vi "Main.vi"() -> ()   [LabVIEW 2018]
uses:
  Ctl/State.ctl
  Ctl/TriggerType.ctl
  Ctl/AO Channel.ctl
  <vilib>/DAQmx/write.llb/DAQmx Write (Digital 1D Bool NChan 1Samp 1Line).vi
  <vilib>/DAQmx/read.llb/DAQmx Read (Digital 1D Bool NChan 1Samp 1Line).vi
  <vilib>/DAQmx/read.llb/DAQmx Read (Analog 1D DBL NChan 1Samp).vi
  <vilib>/DAQmx/write.llb/DAQmx Write (Analog 1D DBL NChan 1Samp).vi
  <vilib>/DAQmx/miscellaneous.llb/DAQmx Fill In Error Info.vi
  Global Variable/StorageAcquireData.vi
panel:
  out "不响应修改预设波形":bool
  out "电流方向":string
  in  "电流反向输出":bool
  in  "电流正向输出":bool=TRUE
  out "电流方向开关输出":bool[](array[boolean])
  out "数字信号错误输出":errorcluster
  in  "数字输出通道参数设置":T1={"数据输出通道设置"={"lines"="", "line grouping"=1}, "采样设置"={"rate"=1000.0, "sample mode"=10178, "samples per channel"=1000}, "ConvLateErrorsToWarnings"=FALSE} {"采样设置"."sample mode" items=["Finite Samples"=10178, "Continuous Samples"=10123, "Hardware Timed Single Point"=12522]; "采样设置"."rate" format="%0.2f"; "数据输出通道设置"."line grouping" items=["one channel for each line", "one channel for all lines"]}
  in  "DAQ数字采集通道参数设置":T2={"数据采集设置"={"lines"="", "line grouping"=1}, "采样设置"={"rate"=1000.0, "sample mode"=10178, "samples per channel"=1000}, "ConvLateErrorsToWarnings"=FALSE} {"采样设置"."sample mode" items=["Finite Samples"=10178, "Continuous Samples"=10123, "Hardware Timed Single Point"=12522]; "采样设置"."rate" format="%0.2f"; "数据采集设置"."line grouping" items=["one channel for each line", "one channel for all lines"]}
  in  "模拟输出通道设置":T3={"数据输出通道设置"={"maximum value"=5.0, "minimum value"=-5.0, "input terminal configuration"=-1, "physical channels"=""}, "采样设置"={"rate"=1000.0, "sample mode"=10178, "samples per channel"=1000}, "ConvLateErrorsToWarnings"=FALSE} {"采样设置"."sample mode" items=["Finite Samples"=10178, "Continuous Samples"=10123, "Hardware Timed Single Point"=12522]; "采样设置"."rate" format="%0.2f"; "数据输出通道设置"."input terminal configuration" items=["Default"=-1, "RSE"=10083, "NRSE"=10078, "Differential"=10106, "Pseudodifferential"=12529]; "数据输出通道设置"."minimum value" format="%0.2f"; "数据输出通道设置"."maximum value" format="%0.2f"}
  in  "DAQ模拟采集通道参数设置":T4={"数据采集通道设置"={"physical channels"="", "maximum value"=5.0, "minimum value"=-5.0, "input terminal configuration"=-1}, "采样设置"={"rate"=1000.0, "sample mode"=10178, "samples per channel"=1000}, "ConvLateErrorsToWarnings"=FALSE} {"采样设置"."sample mode" items=["Finite Samples"=10178, "Continuous Samples"=10123, "Hardware Timed Single Point"=12522]; "采样设置"."rate" format="%0.2f"; "数据采集通道设置"."input terminal configuration" items=["Default"=-1, "RSE"=10083, "NRSE"=10078, "Differential"=10106, "Pseudodifferential"=12529]; "数据采集通道设置"."minimum value" format="%0.2f"; "数据采集通道设置"."maximum value" format="%0.2f"}
  out "预设电流波形":cluster{"xi used":dbl[], "yi":dbl[]}(graph)
  out "插值后输出波形幅值":dbl[](array[numeric])
  in  "修改波形参数":T5
  in  "导入导出波形文件":T6
  in  "预设波形数组":dbl[][](array[numeric])
  out "波形解析成功":bool
  in  "一炮最长运行时间点（ms)":dbl
  in  "PID 参数":T7={"proportional gain (Kc)"=1.0, "integral time (Ti, min)"=0.01, "derivative time (Td, min)"=0.0} {"derivative time (Td, min)" format="%.3f"; "integral time (Ti, min)" format="%.3f"; "proportional gain (Kc)" format="%.3f"}
  in  "触发时间":dbl
  out "模拟信号错误":errorcluster caption="模拟信号错误输出"
  in  "READY_COLD_TO_HOT":bool=TRUE
  out "电源下一个状态":T8
  out "程序停止":bool
  in  "停止":bool
  in  "外部故障":bool
  out "故障状态指示":cluster{"模拟信号故障？":bool, "数字信号故障？":bool}
  in  "模拟保护信号设定值":cluster{"设定值":dbl, "保护配置规则":bool}
  in  "触发参数设置":cluster{"枚举":T9, "触发基准电平":dbl}
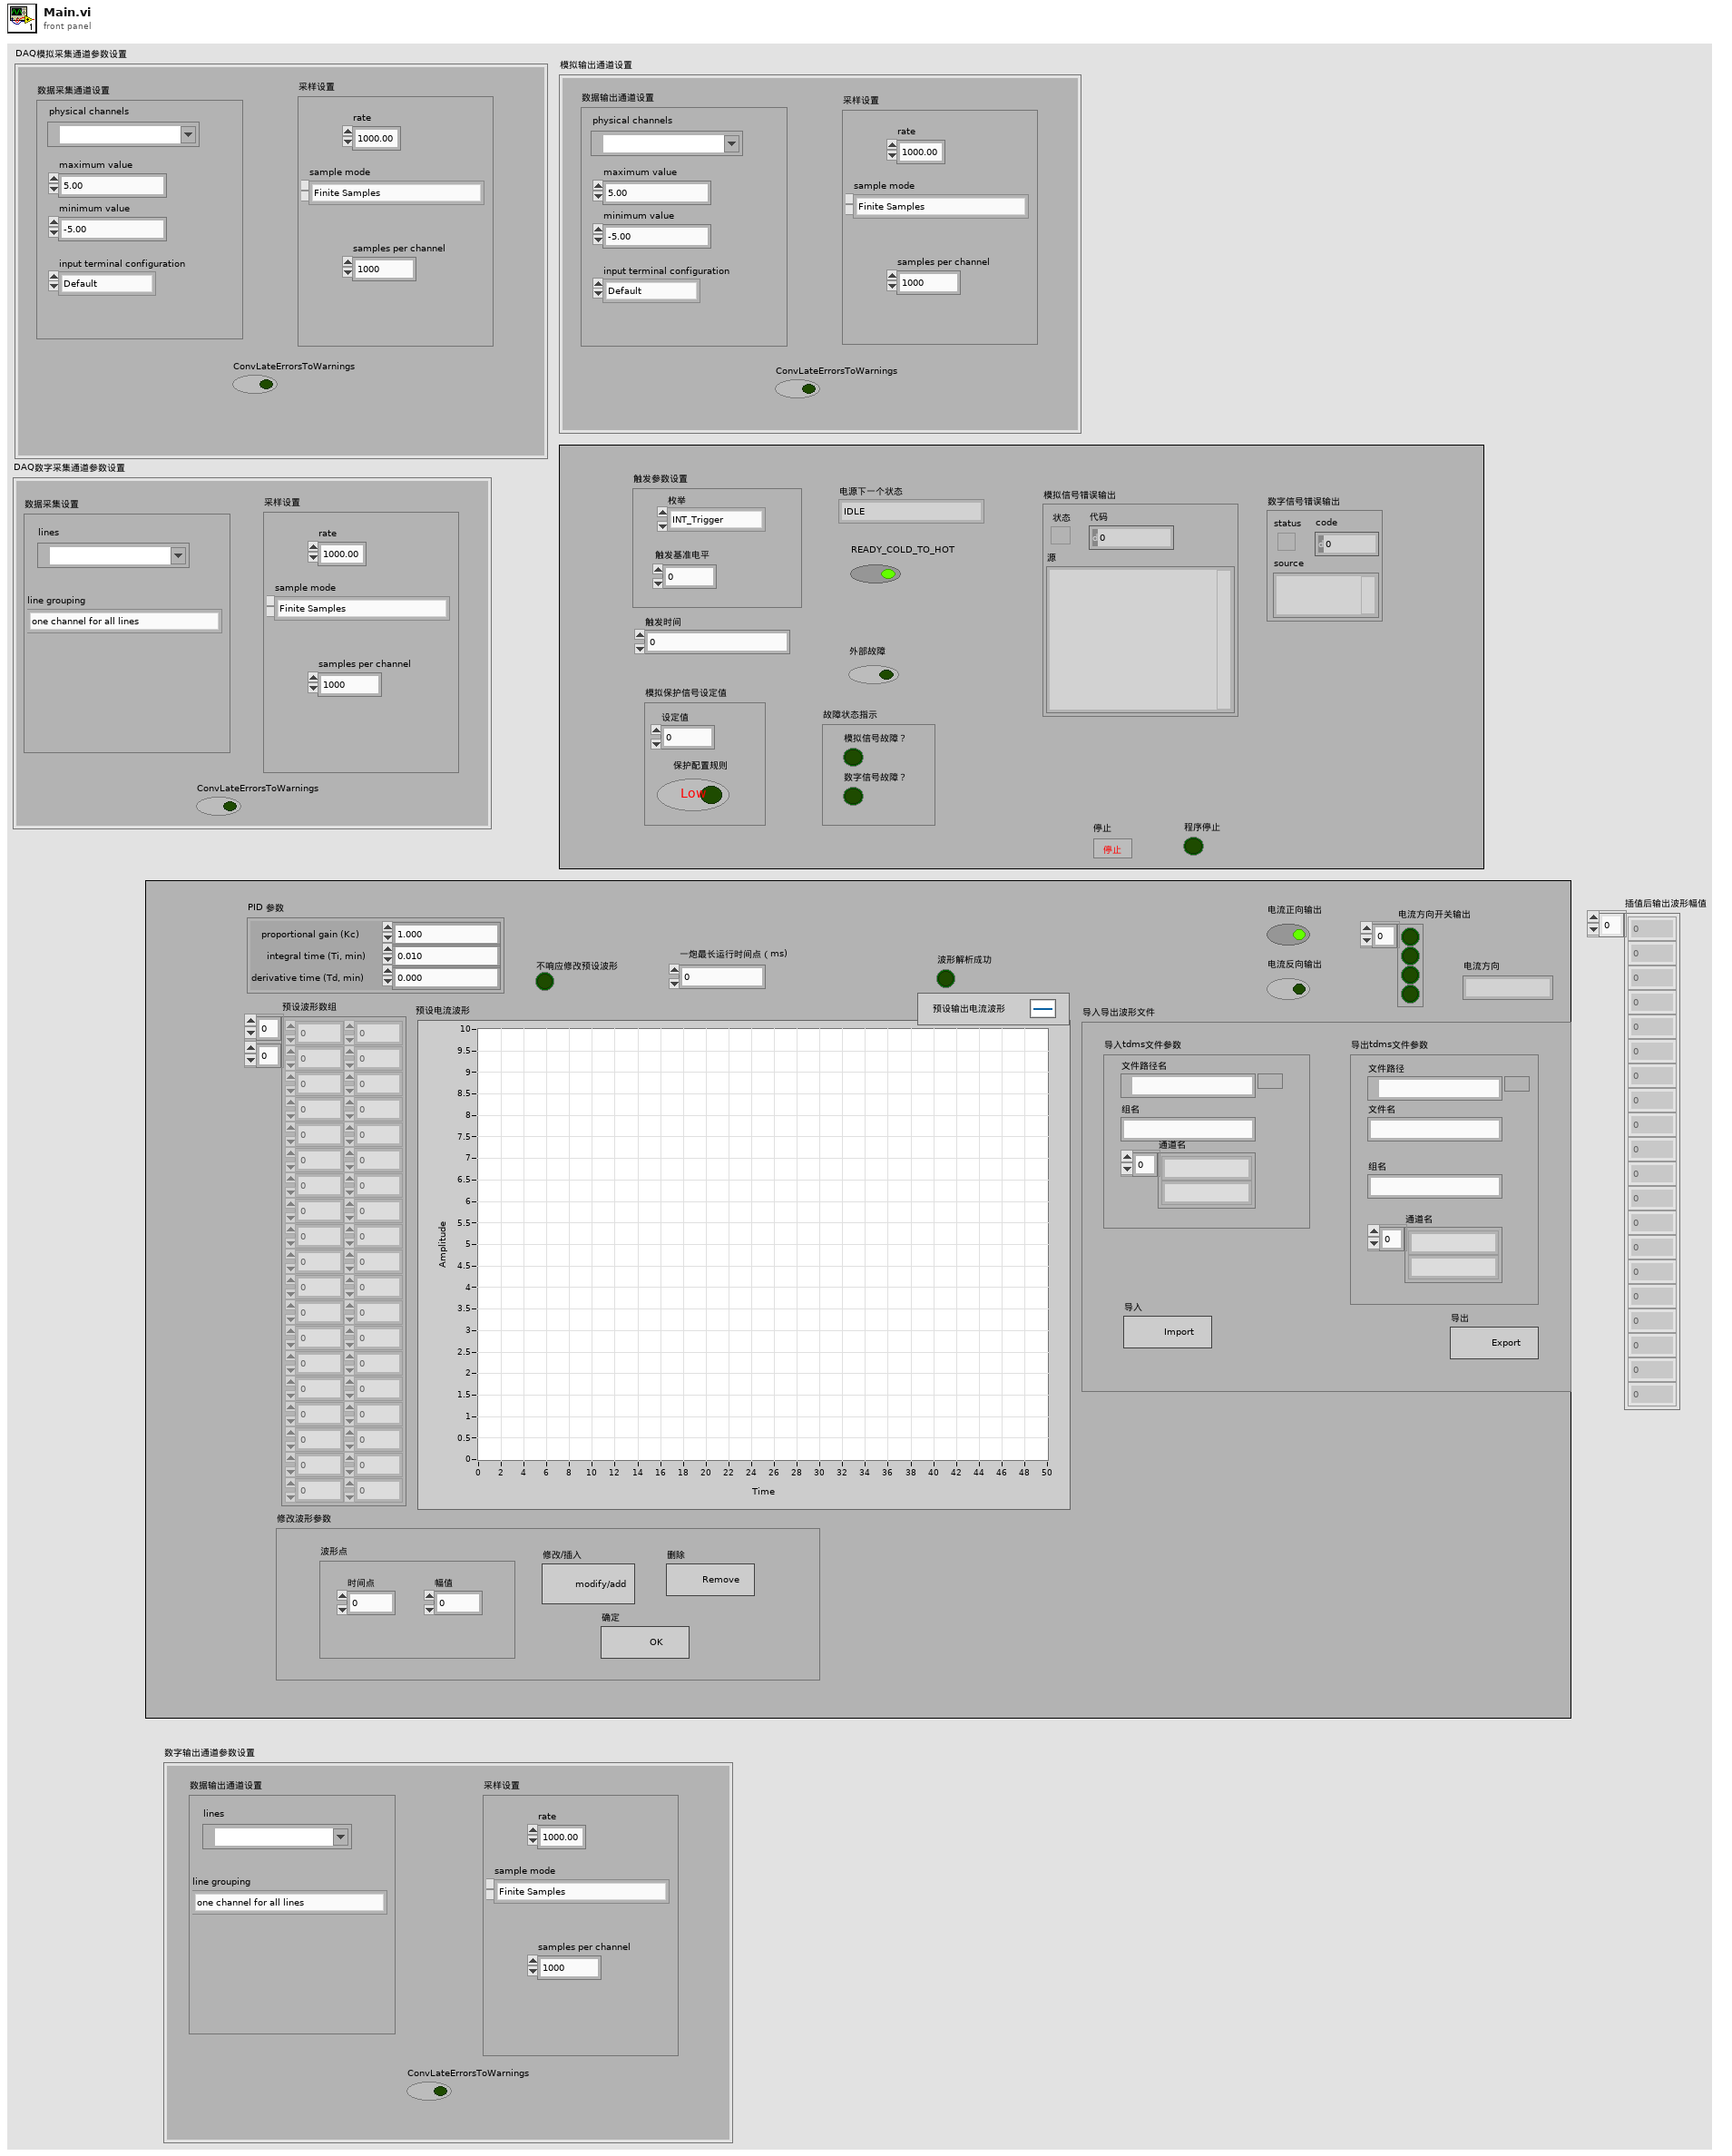
[diagram p1: front panel]
types:
  T1 = cluster{"数据输出通道设置":cluster{"lines":tag, "line grouping":i32}, "采样设置":cluster{"rate":dbl, "sample mode":i32, "samples per channel":i32}, "ConvLateErrorsToWarnings":bool}
  T2 = cluster{"数据采集设置":cluster{"lines":tag, "line grouping":i32}, "采样设置":cluster{"rate":dbl, "sample mode":i32, "samples per channel":i32}, "ConvLateErrorsToWarnings":bool}
  T3 = cluster{"数据输出通道设置":cluster{"maximum value":dbl, "minimum value":dbl, "input terminal configuration":i32, "physical channels":tag}, "采样设置":cluster{"rate":dbl, "sample mode":i32, "samples per channel":i32}, "ConvLateErrorsToWarnings":bool}
  T4 = cluster{"数据采集通道设置":cluster{"physical channels":tag, "maximum value":dbl, "minimum value":dbl, "input terminal configuration":i32}, "采样设置":cluster{"rate":dbl, "sample mode":i32, "samples per channel":i32}, "ConvLateErrorsToWarnings":bool}
  T5 = cluster{"波形点":cluster{"时间点":dbl, "幅值":dbl}, "修改/插入":bool, "删除":bool, "确定":bool}
  T6 = cluster{"导出tdms文件参数":cluster{"组名":string, "通道名":string[], "文件路径":path, "文件名":string}, "导入tdms文件参数":cluster{"文件路径名":path, "组名":string, "通道名":string[]}, "导入":bool, "导出":bool}
  T7 = cluster{"proportional gain (Kc)":dbl, "integral time (Ti, min)":dbl, "derivative time (Td, min)":dbl}
  T8 = typedef "State.ctl" = enum16{"IDLE", "READY_COLD", "READY_HOT", "RUN", "ERROR"}
  T9 = typedef "TriggerType.ctl" = enum16{"INT_Trigger", "Ext_Trigger"}
  T10 = typedef "AO Channel.ctl" = enum16{"启用1个输出通道", "启用2个输出通道", "启用3个输出通道", "启用4个输出通道", "启用5个输出通道", "启用6个输出通道", "启用7个输出通道", "启用8个输出通道"}
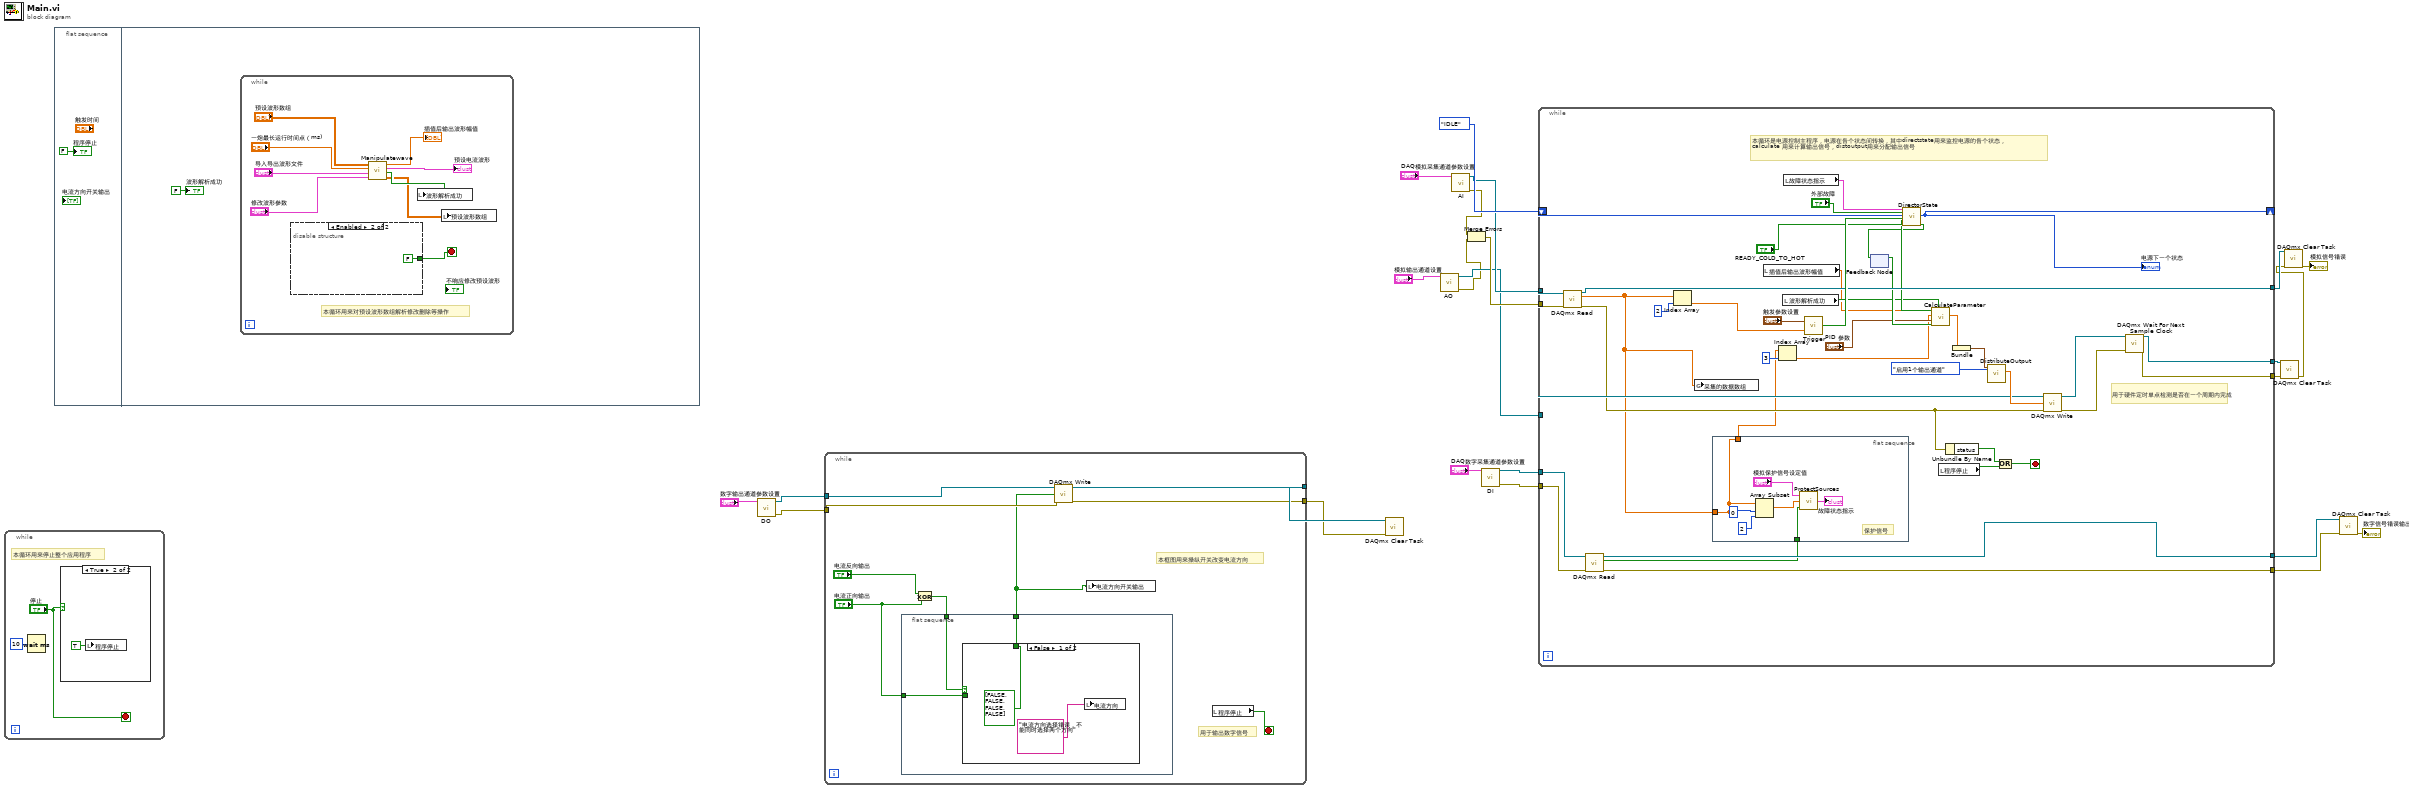
[diagram p0: block diagram]
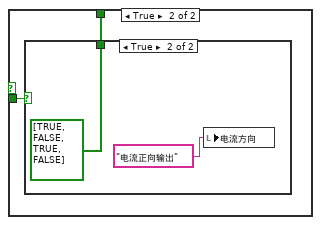
[diagram p2: hidden frame]
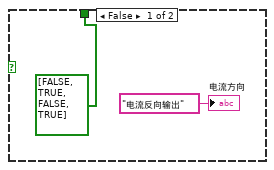
[diagram p3: hidden frame]
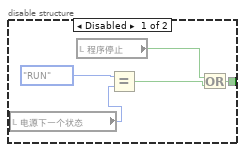
[diagram p4: hidden frame]
diagram:
  n1 = while {
    stop <- "停止" stop-if-true
    # "本循环用来停止整个应用程序"
    n2 = Wait (ms)(milliseconds to wait=u32 10) -> ()  [unwired: 1 out]
    n3 = case shown="True" "停止" {
      frame False {
      }
      frame True {
        n4 = local write "程序停止"(TRUE ("布尔")) -> ()
      }
    }
  }
  n5 = flat-sequence {
    frame #0 {
      "程序停止" <- FALSE ("布尔")
    }
    frame #1 {
      n6 = while {
        stop <- w31 stop-if-true
        # "本循环用来对预设波形数组解析修改删除等操作"
        n7 = disable-structure shown="Enabled" {
          disable-tunnel: [w39 FALSE] -> w31
          frame Disabled {
            n8 = local read "电源下一个状态"() -> (w43:T8)
            n9 = local read "程序停止"() -> (w41:bool)
            n10 = Equal?(x=State."RUN" ("电源状态"), y=w43) -> (x = y?=w40:bool)
            n11 = Or(x=w41, y=w40) -> (x .or. y?=w39:bool)
          }
          frame Enabled {
          }
        }
        n12 = call "Manipulatewave.vi"("修改波形参数"="修改波形参数", "导入导出波形文件"="导入导出波形文件", "一炮最长运行时间点（ms)"="一炮最长运行时间点（ms)", "预设波形数组"="预设波形数组") -> ("波形数组"=w30:dbl[][], "波形解析正确"=w32:bool, "XY Graph"=→"预设电流波形":cluster{"xi used":dbl[], "yi":dbl[]}, "插值后输出波形幅值"=→"插值后输出波形幅值":dbl[])  [unwired: 4 in]
        n13 = local write "波形解析成功"(w32) -> ()
        n14 = local write "预设波形数组"(w30) -> ()
      }
      "波形解析成功" <- FALSE ("波形解析成功")
    }
  }
  n15 = call "DO.vi"("数字输出通道参数设置"="数字输出通道参数设置") -> ("error out"=w1:errorcluster, "task out"=w2:refnum<k21>)  [unwired: 9 in]
  n16 = while {
    tunnel: [w52] -> w4
    tunnel: [w51] -> w3
    tunnel: w2 -> [w50]
    tunnel: w1 -> [w49]
    stop <- w53 stop-if-true
    # "本框图用来操纵开关改变电流方向"
    # "用于输出数字信号"
    n17 = flat-sequence {
      tunnel: w47 -> [w56]
      tunnel: "电流正向输出" -> [w55]
      tunnel: [w54] -> w45
      frame #0 {
        n18 = case shown="False" w56 {
          tunnel: w55 -> [_ w60]
          tunnel: [bool[] [FALSE, FALSE, FALSE, FALSE] ("电流方向开关输出") w59] -> w54
          frame False {
            n19 = local write "电流方向"("电流方向选择错误，不能同时选择两个方向" ("电流方向")) -> ()
          }
          frame True {
            n20 = case shown="True" w60 {
              tunnel: [bool[] [FALSE, TRUE, FALSE, TRUE] ("电流方向开关输出") bool[] [TRUE, FALSE, TRUE, FALSE] ("电流方向开关输出")] -> w59
              frame False {
                "电流方向" <- "电流反向输出" ("电流方向")
              }
              frame True {
                n21 = local write "电流方向"("电流正向输出" ("电流方向")) -> ()
              }
            }
          }
        }
      }
    }
    n22 = Exclusive Or(1:"电流正向输出", 2:"电流反向输出") -> (0:w47:bool)
    n23 = call-poly <vilib>:"DAQmx Write.vi"("task/channels in"=w50, "data"=w45, "error in"=w49) -> ("task out"=w52:refnum<k21>, "error out"=w51:errorcluster)  [unwired: 10 in, 1 out]
    n24 = local write "电流方向开关输出"(w45) -> ()
    n25 = local read "程序停止"() -> (w53:bool)
  }
  n26 = call <vilib>:"DAQmx Clear Task.vi"("task in"=w4, "error in"=w3) -> ()  [unwired: 13 in, 1 out]
  n27 = call "AO.vi"("模拟输出通道设置"="模拟输出通道设置") -> ("error out"=w12:errorcluster, "task out"=w13:refnum<k21>)  [unwired: 8 in]
  n28 = call "AI.vi"("DAQ模拟采集通道参数设置"="DAQ模拟采集通道参数设置") -> ("error out"=w16:errorcluster, "task out"=w15:refnum<k21>)  [unwired: 8 in]
  n29 = Merge Errors(w16, w12) -> (w23:errorcluster)
  n30 = call "DI.vi"("DAQ数字采集通道参数设置"="DAQ数字采集通道参数设置") -> ("error out"=w9:errorcluster, "task out"=w10:refnum<k21>)  [unwired: 9 in]
  n31 = while {
    shift-right: [w103] -> _
    shift-left: State."IDLE" ("电源状态") -> [w104]
    tunnel: w15 -> [w99]
    tunnel: w23 -> [w98]
    tunnel: w13 -> [w89]
    tunnel: [w86] -> w22
    tunnel: [w85] -> w21
    tunnel: [w84] -> w20
    tunnel: w10 -> [w69]
    tunnel: w9 -> [w68]
    tunnel: [w67] -> w8
    tunnel: [w65] -> w7
    stop <- w102 stop-if-true
    # "用于硬件定时单点检测是否在一个周期内完成"
    # "本循环是电源控制主程序，电源在各个状态间转换，其中directstate用来监控电源的各个状态，\ncalculate 用来计算输出信号，distoutput用来分配输出信号"
    n32 = call-poly <vilib>:"DAQmx Read.vi"("task/channels in"=w99, "error in"=w98) -> ("task out"=w84:refnum<k21>, "data"=w70:dbl[], "error out"=w83:errorcluster)  [unwired: 11 in]
    n33 = call-poly <vilib>:"DAQmx Read.vi"("task/channels in"=w69, "error in"=w68) -> ("task out"=w67:refnum<k21>, "data"=w66:bool[], "error out"=w65:errorcluster)  [unwired: 11 in]
    n34 = Index Array(array=w70, index=2) -> (element=w94:dbl)
    n35 = global write "StorageAcquireData.vi" "采集的数据数组"(w70) -> ()
    n36 = flat-sequence {
      tunnel: [w106] -> _
      tunnel: w70 -> [w106]
      tunnel: [w106] -> w71
      tunnel: w66 -> [w105]
      frame #0 {
        # "保护信号"
        n37 = Array Subset(array=w106, index=0, length=2) -> (w107:dbl[])
        n38 = call "ProtectSources.vi"("数字输入保护信号"=w105, "模拟输入保护信号"=w107, "模拟保护信号设定值"="模拟保护信号设定值") -> ("故障状态指示"=→"故障状态指示":cluster{"模拟信号故障？":bool, "数字信号故障？":bool})
      }
    }
    n39 = local read "插值后输出波形幅值"() -> (w72:dbl[])
    n40 = Index Array(array=w71, index=3) -> (element=w74:dbl)
    n41 = local read "波形解析成功"() -> (w73:bool)
    n42 = local read "故障状态指示"() -> (w97:cluster{"模拟信号故障？":bool, "数字信号故障？":bool})
    n43 = call "Trigger.vi"("触发电平"=w94, "触发参数设置"="触发参数设置") -> ("Trigger？"=w93:bool)
    n44 = feedback #1() -> (w79:bool)  [unwired: 1 in]
    n45 = call "CalculateParameter.vi"("波形解析正确"=w73, "enable"=w79, "PID 参数"="PID 参数", "采集的电信号值"=w74, "插值后波形数组"=w72) -> ("输出相关参数"=w78:dbl, "计算模块状态"=w81:bool)  [unwired: 3 in]
    n46 = call "DirectorState.vi"("内部故障"=w97, "外部故障"="外部故障", "电源状态"=w104, "触发状态"=w93, "计算模块状态"=w81, "READY_COLD_TO_HOT"="READY_COLD_TO_HOT") -> ("电源下一个状态"=w103:T8, "enable"=w80:bool)  [unwired: 12 in]
    "电源下一个状态" <- w103
    n47 = feedback-in #1(w80) -> ()
    n48 = local read "程序停止"() -> (w100:bool)
    n49 = Unbundle By Name(w83) -> ("status"=w101:bool)
    n50 = Bundle("输出相关参数"=w78) -> (w77:cluster{"输出相关参数":dbl})  [unwired: 1 in]
    n51 = call "DistributeOutput.vi"("启用输出通道数"=AO_Channel."启用1个输出通道", "一个通道输出AO0"=w77) -> ("输出数组"=w90:dbl[])  [unwired: 9 in]
    n52 = Or(x=w101, y=w100) -> (x .or. y?=w102:bool)
    n53 = call-poly <vilib>:"DAQmx Write.vi"("task/channels in"=w89, "data"=w90, "error in"=w83) -> ("task out"=w87:refnum<k21>, "error out"=w88:errorcluster)  [unwired: 10 in, 1 out]
    n54 = call <vilib>:"DAQmx Wait For Next Sample Clock.vi"("task/channels in"=w87, "error in"=w88) -> ("task out"=w86:refnum<k21>, "error out"=w85:errorcluster)  [unwired: 11 in, 1 out]
  }
  n55 = call <vilib>:"DAQmx Clear Task.vi"("task in"=w22, "error in"=w21) -> ("error out"=w19:errorcluster)  [unwired: 13 in]
  n56 = call <vilib>:"DAQmx Clear Task.vi"("task in"=w20, "error in"=w19) -> ("error out"=→"模拟信号错误":errorcluster)  [unwired: 13 in]
  n57 = call <vilib>:"DAQmx Clear Task.vi"("task in"=w8, "error in"=w7) -> ("error out"=→"数字信号错误输出":errorcluster)  [unwired: 13 in]
